vi "execution.vi"() -> ()   [LabVIEW 2018]
doc: "You can use the System Exec VI to call command line utilities that return standard output to the command shell. You also can call interactive applications that you intend to launch using System Exec, but interact with using the UI of the executable."
panel:
  out "standard output":string
  out "standard error":string
  out "return code":i32
  # "Overview: Demonstrates a way to use the System Exec VI to programmatically run and pass parameters to run PhaseSpace program.\nRequirements: Windows"
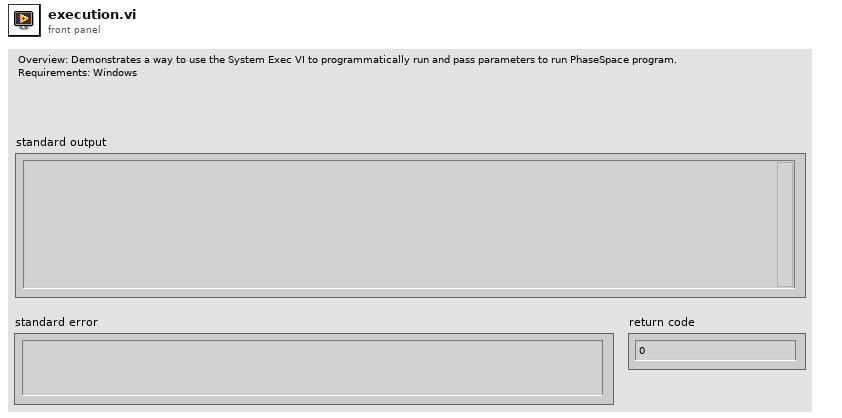
[diagram p1: front panel]
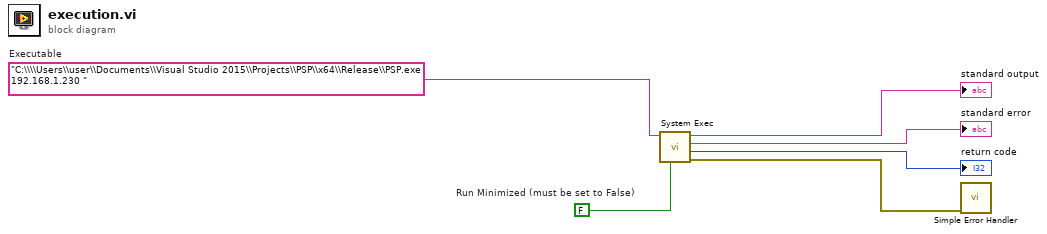
[diagram p0: block diagram]
diagram:
  w1 = FALSE  # Run Minimized (must be set to False)
  w6 = "C:\\\\Users\\user\\Documents\\Visual Studio 2015\\Projects\\PSP\\x64\\Release\\PSP.exe 192.168.1.230 "  # Executable
  n1 = call <vilib>:"System Exec.vi"("run minimized? (F)"=w1, "command line"=w6) -> ("error out"=w2:errorcluster, "return code"=→"return code":i32, "standard error"=→"standard error":string, "standard output"=→"standard output":string)  [unwired: 6 in]
  n2 = call <vilib>:"Simple Error Handler.vi"("error in (no error)"=w2) -> ()  [unwired: 1 in, 8 out]
